vi "Pulse DIO Line Script.vi"(7 "port number (0)":u8, 8 "error in (no error)":errorcluster, 9 "DIO line number (0)":u8, 10 "pulse width delay [ms] (0)":u8, 11 "spi script reference in":T1) -> (0 "error out":errorcluster, 3 "spi script reference out":T1)   [LabVIEW 2013]
doc: "Pulses the given DIO line high then low with pulse width and preceding delay time given by pulse width delay."
uses:
  <vilib>/ni845x/ni845x.llb/ni845xSpiScriptControl.ctl
  <vilib>/ni845x/ni845x.llb/ni845xDioLineWriteValue.ctl
  <vilib>/ni845x/ni845x.llb/NI-845x SPI Script Ms Delay.vi
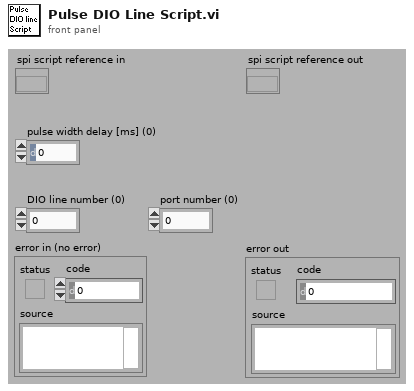
[diagram p1: front panel]
types:
  T1 = typedef "ni845xSpiScriptControl.ctl" = refnum<k20>
  T2 = typedef "ni845xDioLineWriteValue.ctl" = i32
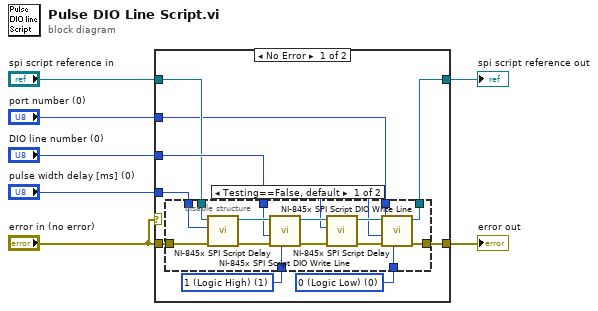
[diagram p0: block diagram]
diagram:
  n1 = case shown="No Error" "error in (no error)" {
    tunnel: [w16 w34] -> w7
    tunnel: [w15 w35] -> w6
    tunnel: "error in (no error)" -> [w12 w35]
    tunnel: "pulse width delay [ms] (0)" -> [w11 _]
    tunnel: "DIO line number (0)" -> [w10 _]
    tunnel: "spi script reference in" -> [w9 w34]
    tunnel: "port number (0)" -> [w8 _]
    frame No Error {
      w14 = T2 1 items=["0 (Logic Low)", "1 (Logic High)"] ("write value")
      w13 = T2 0 items=["0 (Logic Low)", "1 (Logic High)"] ("write value")
      n2 = disable-structure shown="Testing==False, default" {
        disable-tunnel: [w25 w33] -> w16
        disable-tunnel: [w24 w32] -> w15
        disable-tunnel: w14 -> [w23 _]
        disable-tunnel: w13 -> [w22 _]
        disable-tunnel: w12 -> [w21 w32]
        disable-tunnel: w11 -> [w20 _]
        disable-tunnel: w10 -> [w19 _]
        disable-tunnel: w9 -> [w18 w33]
        disable-tunnel: w8 -> [w17 _]
        frame condition #0 (active) {
          n3 = call-poly <vilib>:"NI-845x SPI Script Delay.vi"("error in (no error)"=w21, "delay in milliseconds (0)"=w20, "spi script reference in"=w18) -> ("error out"=w26:errorcluster, "spi script reference out"=w27:T1)  [unwired: 7 in]
          n4 = call <vilib>:"NI-845x SPI Script DIO Write Line.vi"("write value"=w23, "error in (no error)"=w26, "line number (0)"=w19, "spi script reference in"=w27) -> ("error out"=w29:errorcluster, "spi script reference out"=w28:T1)  [unwired: 6 in]
          n5 = call-poly <vilib>:"NI-845x SPI Script Delay.vi"("error in (no error)"=w29, "delay in milliseconds (0)"=w20, "spi script reference in"=w28) -> ("error out"=w31:errorcluster, "spi script reference out"=w30:T1)  [unwired: 7 in]
          n6 = call <vilib>:"NI-845x SPI Script DIO Write Line.vi"("write value"=w22, "error in (no error)"=w31, "line number (0)"=w19, "port number (0)"=w17, "spi script reference in"=w30) -> ("error out"=w24:errorcluster, "spi script reference out"=w25:T1)  [unwired: 5 in]
        }
        frame condition #1 {
        }
      }
    }
    frame Error {
    }
  }
  "spi script reference out" <- w7
  "error out" <- w6
